vi "Pulso_se_Mudou.vi"(1 "Entrada":bool) -> (0 "Saída":bool)   [LabVIEW 2018]
panel:
  in  "AUX MUDA":bool
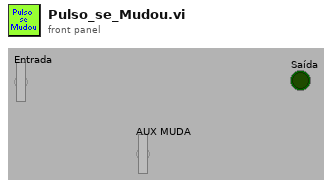
[diagram p1: front panel]
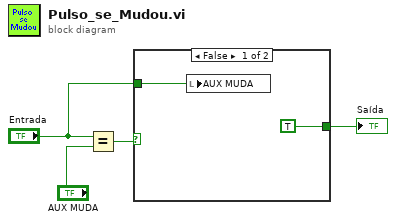
[diagram p0: block diagram]
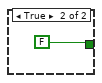
[diagram p2: hidden frame]
diagram:
  n1 = Equal?(x="Entrada", y="AUX MUDA") -> (x = y?=w3:bool)
  n2 = case shown="False" w3 {
    tunnel: "Entrada" -> [w6 _]
    tunnel: [TRUE FALSE] -> w1
    frame False {
      n3 = local write "AUX MUDA"(w6) -> ()
    }
    frame True {
    }
  }
  "Saída" <- w1
